vi "HB Noise Threshold.vi"(8 "Error In":errorcluster, 10 "p":i32, 11 "Y":dbl[](array[numeric])) -> (0 "Error Out":errorcluster, 2 "R2":dbl, 3 "P":dbl)   [LabVIEW 2017, in "Math Utilities.lvlib"]
doc: "<B>HB Noise Threshold</B> determines the noise threshold for a given signal on a fixed frequency range. The algorithm is based on Hildebrand and Sekhon [1974]. Data is first ordered in descending order. Then, each point is tested until R2 >= 1 at which point the routine exits with a given noise threshold <B>P</B>."
uses:
  Math Utilities.lvlib
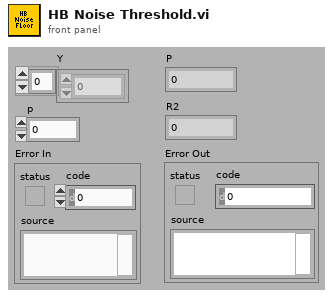
[diagram p1: front panel]
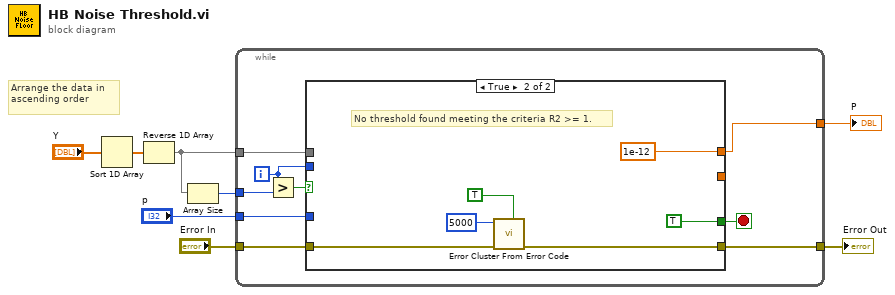
[diagram p0: block diagram]
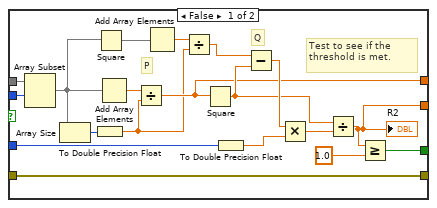
[diagram p2: hidden frame]
diagram:
  # "Arrange the data in ascending order"
  n1 = Sort 1D Array(array="Y") -> (sorted array=w3:dbl[])
  n2 = Reverse 1D Array(array=w3) -> (reversed array=w2:dbl[])
  n3 = Array Size(array=w2) -> (size(s)=w5:i32)
  n4 = while {
    tunnel: w2 -> [w17]
    tunnel: w5 -> [w14]
    tunnel: [w13] -> w6
    tunnel: "Error In" -> [w12]
    tunnel: [w10] -> w4
    tunnel: "p" -> [w9]
    i -> [w15]
    stop <- w11 stop-if-true
    n5 = Greater?(x=w15, y=w14) -> (0:w16:bool)
    n6 = case shown="True" w16 {
      tunnel: w17 -> [w36 _]
      tunnel: w15 -> [w35 _]
      tunnel: [w24 TRUE] -> w11
      tunnel: [w26 w40] -> w13
      tunnel: w12 -> [w26 w41]
      tunnel: [w25 1e-12] -> w10
      tunnel: [w23 _] -> _
      tunnel: w9 -> [w18 _]
      frame False {
        # "Test to see if the threshold is met."
        # "Q"
        # "P"
        n7 = Array Subset(array=w36, index=w35) -> (w22:dbl[])  [unwired: 1 in]
        n8 = Array Size(array=w22) -> (size(s)=w21:i32)
        n9 = To Double Precision Float(number=w21) -> (double precision float=w20:dbl)
        n10 = Square(x=w22) -> (x^2=w33:dbl[])
        n11 = Add Array Elements(numeric array=w22) -> (sum=w34:dbl)
        n12 = Divide(x=w34, y=w20) -> (x/y=w25:dbl)
        n13 = Add Array Elements(numeric array=w33) -> (sum=w32:dbl)
        n14 = Divide(x=w32, y=w20) -> (x/y=w31:dbl)
        n15 = Square(x=w25) -> (x^2=w28:dbl)
        n16 = To Double Precision Float(number=w18) -> (double precision float=w19:dbl)
        n17 = Subtract(x=w31, y=w28) -> (x-y=w30:dbl)
        n18 = Multiply(x=w30, y=w19) -> (x*y=w29:dbl)
        n19 = Divide(x=w28, y=w29) -> (x/y=w23:dbl)
        "R2" <- w23
        n20 = Greater Or Equal?(x=w23, y=1.0) -> (x >= y?=w24:bool)
      }
      frame True {
        # "No threshold found meeting the criteria R2 >= 1."
        n21 = call <vilib>:"Error Cluster From Error Code.vi"("is warning? (False)"=TRUE, "error in (no error)"=w41, "error code (0)"=5000) -> ("error out"=w40:errorcluster)  [unwired: 1 in, 5 out]
      }
    }
  }
  "Error Out" <- w6
  "P" <- w4
